vi "Set Exp_tmp.vi"(8 "error in (no error)":errorcluster, 9 "Copy only data":bool, 10 "Experiment.lvclass":refnum<class "Experiment.lvclass">, 11 "Control-Client in":refnum<class "Control-Client.lvclass">) -> (0 "error out":errorcluster, 3 "Control-Client out":refnum<class "Control-Client.lvclass">)   [LabVIEW 2015, in "Control-Client.lvclass"]
uses:
  Control-Client.lvclass
  Experiments/Experiment.lvclass
  Control-Client.lvclass/Control-Client.ctl
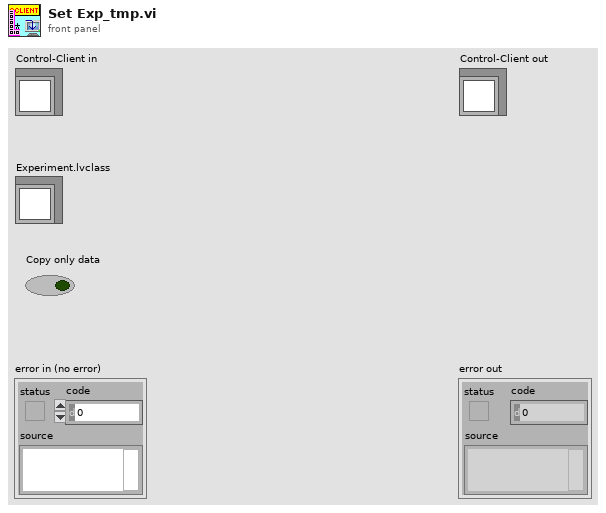
[diagram p1: front panel]
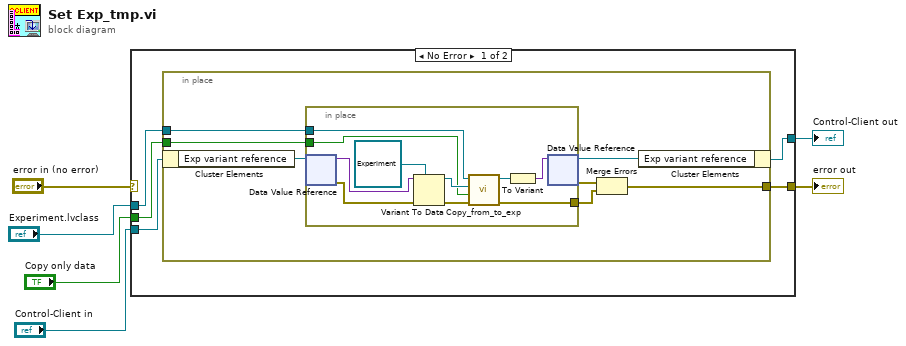
[diagram p0: block diagram]
diagram:
  n1 = case shown="No Error" "error in (no error)" {
    selector: "error in (no error)" -> [_ w30]
    tunnel: [w11 w30] -> w5
    tunnel: [w8 w29] -> w3
    tunnel: "Control-Client in" -> [w9 w29]
    tunnel: "Experiment.lvclass" -> [w10 _]
    tunnel: "Copy only data" -> [w7 _]
    frame No Error {
      n2 = in-place {
        in-place-border: [w18] -> w11
        in-place-border: w10 -> [w13]
        in-place-border: w7 -> [w12]
        n3 = in-place-cluster #1(w9) -> ("Exp variant reference"=w17:refnum<data-value>)
        n4 = in-place {
          in-place-border: [w20] -> w15
          in-place-border: w13 -> [w24]
          in-place-border: w12 -> [w19]
          n5 = in-place-dvr #2(w17) -> (w26:variant, w28:errorcluster)
          n6 = Variant To Data(error in=w28, type=refnum<class "Experiment.lvclass"> refnum ("Experiment.lvclass"), Variant=w26) -> (data=w25:refnum<class "Experiment.lvclass">, error out=w23:errorcluster)
          n7 = call "Copy_from_to_exp.vi"("error in (no error)"=w23, "Copy only data"=w19, "Experiment copy to"=w25, "Experiment copy from"=w24) -> ("error out"=w20:errorcluster, "Experiment copied"=w22:refnum<class "Experiment.lvclass">)  [unwired: 6 in]
          n8 = To Variant(anything=w22) -> (Variant=w21:variant)
          n9 = in-place-dvr #2(w21) -> (w16:refnum<data-value>, w14:errorcluster)
        }
        n10 = Merge Errors(w14, w15) -> (w18:errorcluster)
        n11 = in-place-cluster #1("Exp variant reference"=w16) -> (w8:refnum<class "Control-Client.lvclass">)
      }
    }
    frame Error {
    }
  }
  "error out" <- w5
  "Control-Client out" <- w3
